vi "Persistence to Data Type.vi"(8 "error in (no error)":errorcluster, 11 "Persistence":refnum<class "IPersist.lvclass">) -> (0 "error out":errorcluster, 3 "Boolean out":refnum<class "Persistence.lvclass">)   [LabVIEW 2017, in "Custom Type Test Executive.lvlib" / "Persistence.lvclass"]
uses:
  <vilib>/gpm_packages/@cs/test-executive/Source/Custom Type Test Executive/Persistence Data Type/Persistence.lvclass
  <vilib>/gpm_packages/@cs/persistence/source/IPersist/IPersist.lvclass
  <vilib>/gpm_packages/@cs/test-executive/Source/Custom Type Test Executive/Persistence Data Type/Persistence.lvclass/Persistence.ctl
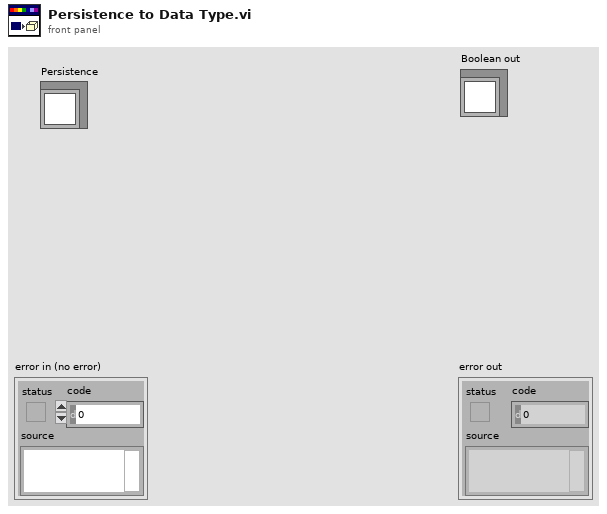
[diagram p1: front panel]
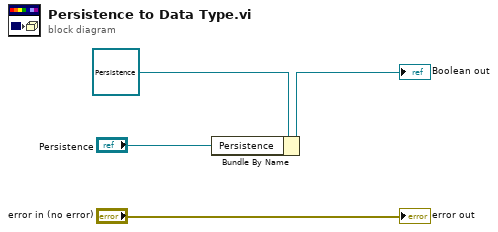
[diagram p0: block diagram]
diagram:
  n1 = Bundle By Name(cluster=refnum<class "Persistence.lvclass"> refnum ("Boolean in"), "Persistence"="Persistence") -> (→"Boolean out":refnum<class "Persistence.lvclass">)
  "error out" <- "error in (no error)"
